vi "Get Data I16_32.vi"(8 "error in (no error)":errorcluster, 11 "Tektronix MSO 6 Driver in":refnum<class "Tektronix MSO 6 Driver.lvclass">) -> (0 "error out":errorcluster, 1 "I32 data out":i32[][](array[numeric]), 2 "I16 data out":i16[][](array[numeric]), 3 "Tektronix MSO 6 Driver out":refnum<class "Tektronix MSO 6 Driver.lvclass">, 4 "Finished":bool, 5 "Current read position":i32)   [LabVIEW 2020, in "Tektronix MSO 6 Driver.lvclass"]
uses:
  Tektronix MSO 6 Driver.lvclass
  C:/GitHub/NHMFL_Core/Libraries/Instruments/Tektronix/Tektronix Driver/Tektronix Driver.lvclass
  C:/GitHub/NHMFL_Core/Libraries/Instruments/Pulse Driver/Pulse Driver.lvclass
  Pulse Driver/Pulse Driver.lvclass/Pulse Driver.ctl
  Pulse Driver/Write dt.vi
  Pulse Driver/Write t0.vi
  Pulse Driver/Write Binary sample width.vi
  <instrlib>/Tektronix MSO5X Series/Tektronix MSO5X Series.lvlib
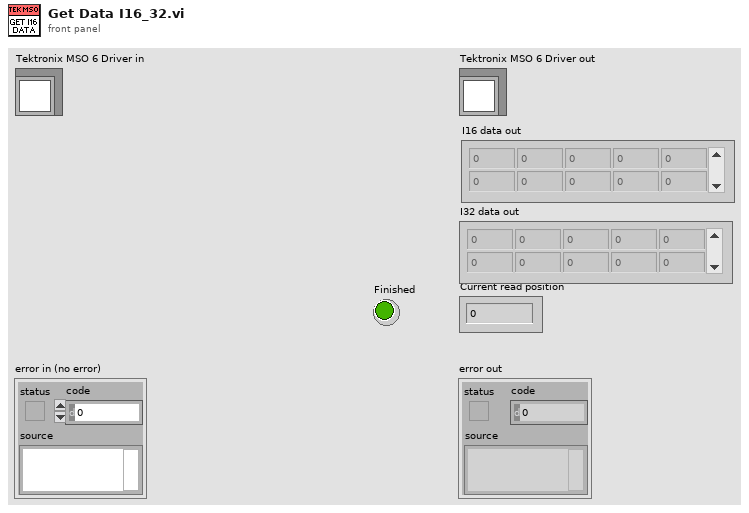
[diagram p1: front panel]
types:
  T1 = typedef "Tektronix Configuration.ctl" = cluster{"Channel":i32, "Number of averages":i32, "Input impedace":enum16{"1 M Ohm", "50 Ohm"}, "Vertical coupling":enum16{"AC", "DC", "Ground"}}
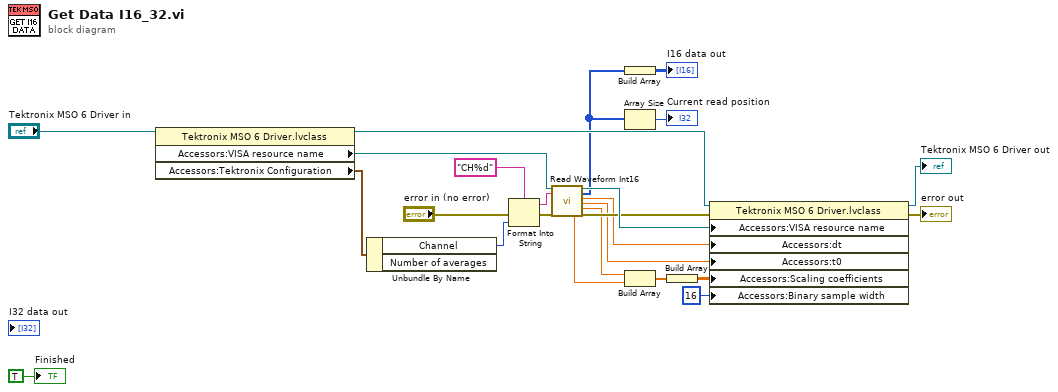
[diagram p0: block diagram]
diagram:
  n1 = property class="Tektronix MSO 6 Driver.lvclass"(reference="Tektronix MSO 6 Driver in") -> (reference out=w21:refnum<class "Tektronix MSO 6 Driver.lvclass">, "Accessors:VISA resource name"=w24:refnum<visa-resource-name>, "Accessors:Tektronix Configuration"=w16:T1)  [unwired: 1 in, 1 out]
  n2 = Unbundle By Name(w16) -> ("Channel"=w17:i32)  [unwired: 1 out]
  n3 = Format Into String(format string="CH%d", error in="error in (no error)", w17) -> (resulting string=w15:string, error out=w13:errorcluster)  [unwired: 1 in]
  n4 = call <instrlib>:"Read Waveform Int16.vi"("VISA resource name"=w24, "Channel (CH1)"=w15, "error in (no error)"=w13) -> ("Scale Factor"=w5:dbl, "VISA resource name out"=w22:refnum<visa-resource-name>, "Waveform Array"=w9:i16[], "X Increment"=w7:dbl, "Initial X Offset"=w1:dbl, "Scale Offset"=w6:dbl, "error out"=w12:errorcluster)  [unwired: 6 in, 4 out]
  n5 = Build Array(w9) -> (→"I16 data out":i16[][])
  n6 = Array Size(array=w9) -> (size(s)=→"Current read position":i32)
  n7 = Build Array(w6, w5) -> (w4:dbl[])
  n8 = Build Array(w4) -> (w3:dbl[][])
  n9 = property class="Tektronix MSO 6 Driver.lvclass"(reference=w21, error in=w12, "Accessors:VISA resource name"=w22, "Accessors:dt"=w7, "Accessors:t0"=w1, "Accessors:Scaling coefficients"=w3, "Accessors:Binary sample width"=16 ("Binary sample width")) -> (reference out=→"Tektronix MSO 6 Driver out":refnum<class "Tektronix MSO 6 Driver.lvclass">, error out=→"error out":errorcluster)
  "Finished" <- TRUE ("Finished")
